vi "Inst_DS360.vi"(8 "error in":errorcluster, 10 "All Message Queues in":T1, 11 "Prueba08 in":refnum<class "Prueba08.lvclass">) -> (0 "error out":errorcluster)   [LabVIEW 2019, in "Prueba08.lvclass"]
uses:
  Prueba08.lvclass
  QMH/Message Queue/All Message Queues.ctl
  QMH/Message Queue/Message Cluster.ctl
  Prueba08.lvclass/Prueba08.ctl
  ClusterGEN.ctl
  <vilib>/Utility/error.llb/Error Cluster From Error Code.vi
  QMH/Message Queue/Enqueue Message (Single).vi
  <vilib>/ErrorRing/Error Ring.xnode
  QMH/Message Queue/Message Queue.lvlib
  Instrumento/DS360/DS360.lvclass
panel:
  out "All States":string[](array[string])
  out "Actual State":string
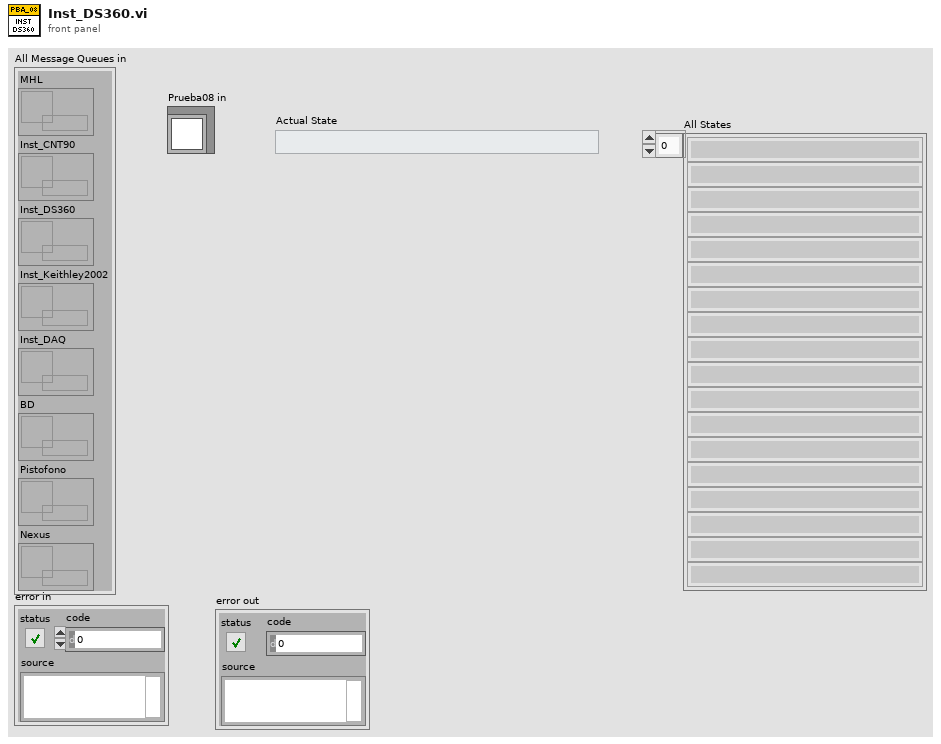
[diagram p1: front panel]
types:
  T1 = typedef "Message Queue.lvlib/All Message Queues.ctl" = cluster{"MHL":refnum<queue>, "Inst_CNT90":refnum<queue>, "Inst_DS360":refnum<queue>, "Inst_Keithley2002":refnum<queue>, "Inst_DAQ":refnum<queue>, "BD":refnum<queue>, "Pistofono":refnum<queue>, "Nexus":refnum<queue>}
  T2 = typedef "Prueba08.lvclass/ClusterGEN.ctl" = cluster{"frec":dbl, "amp":dbl, "ms_burst":dbl}
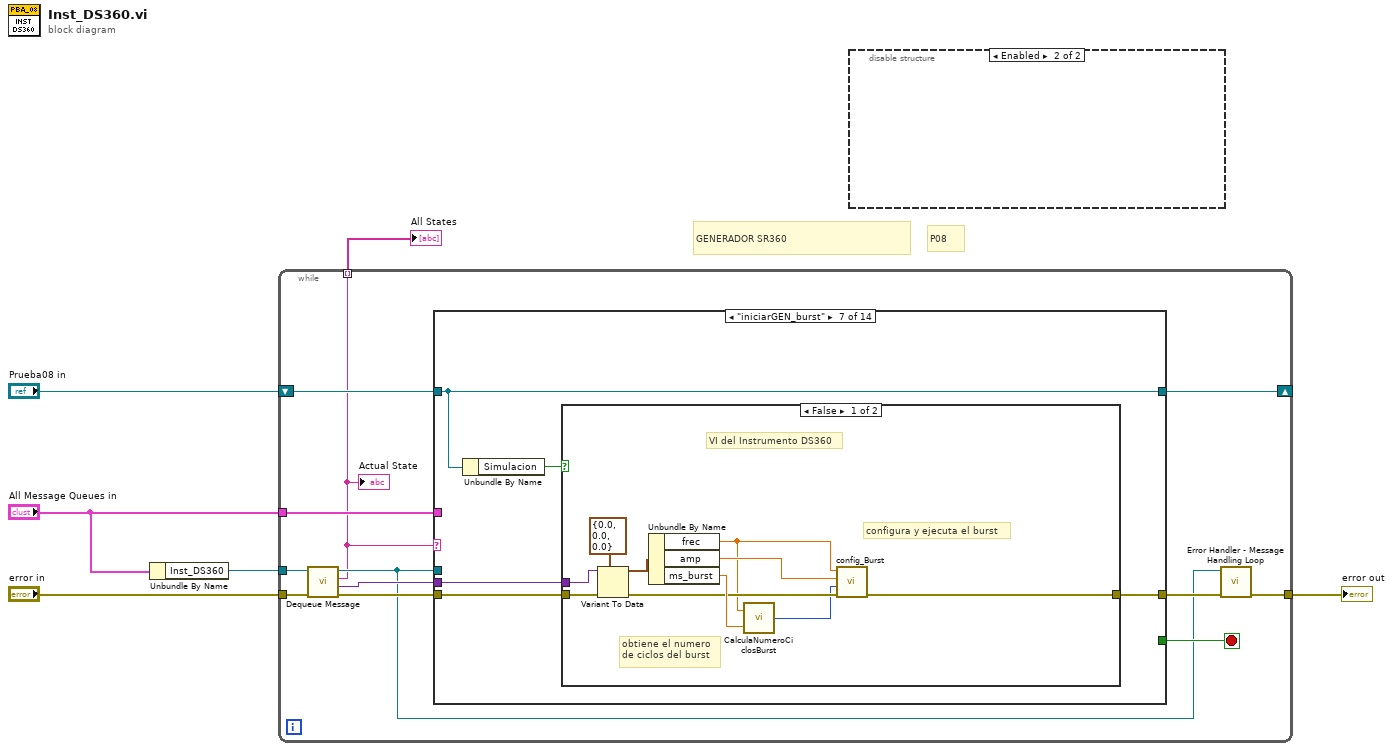
[diagram p0: block diagram]
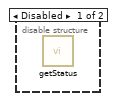
[diagram p2: hidden frame]
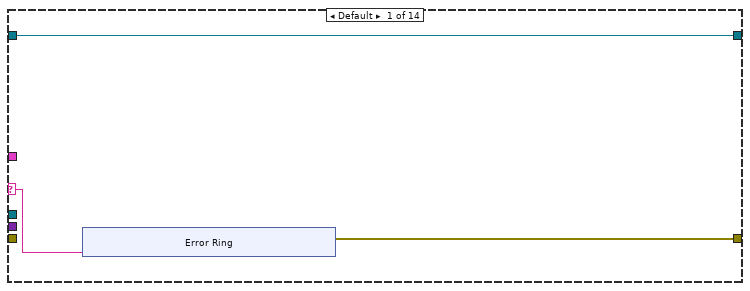
[diagram p3: hidden frame]
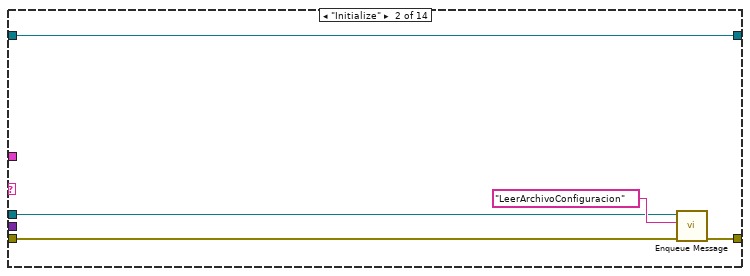
[diagram p4: hidden frame]
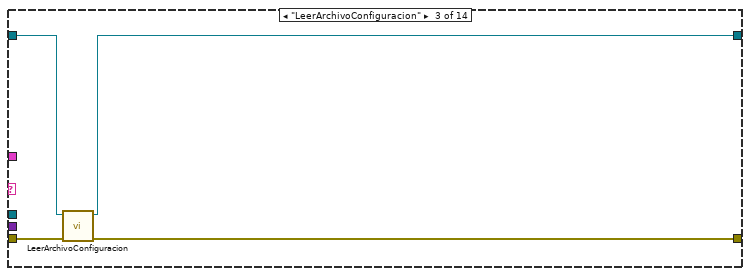
[diagram p5: hidden frame]
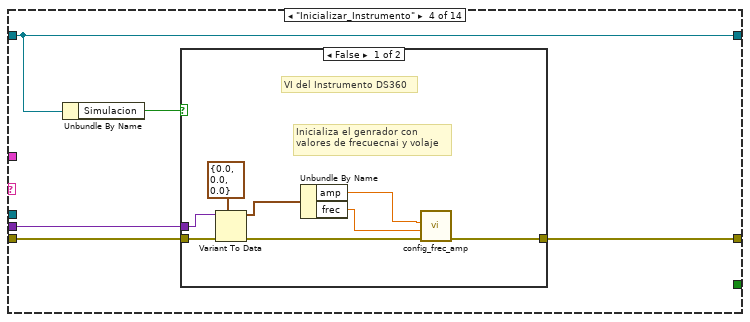
[diagram p6: hidden frame]
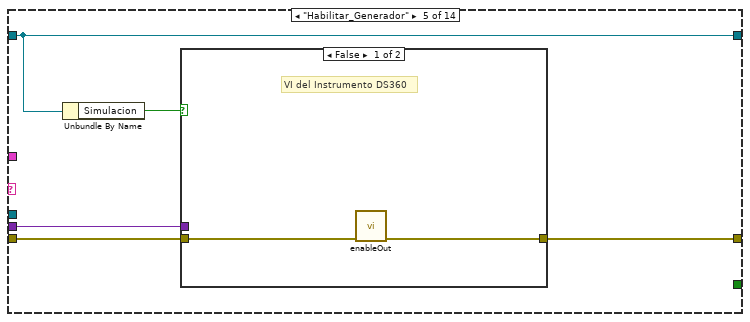
[diagram p8: hidden frame]
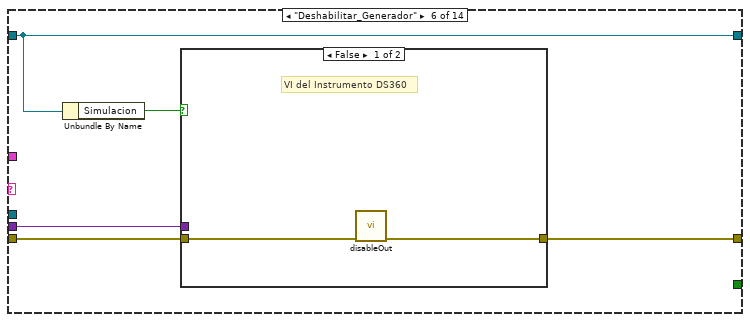
[diagram p10: hidden frame]
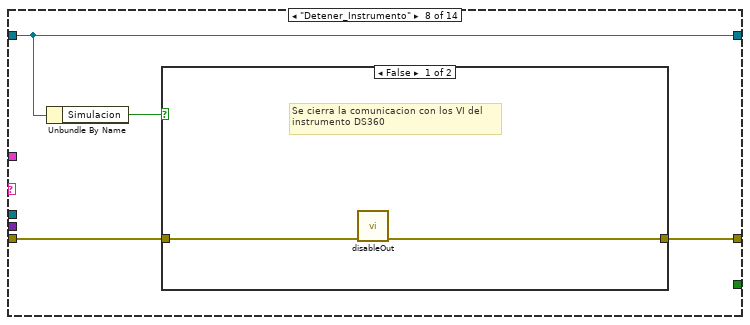
[diagram p13: hidden frame]
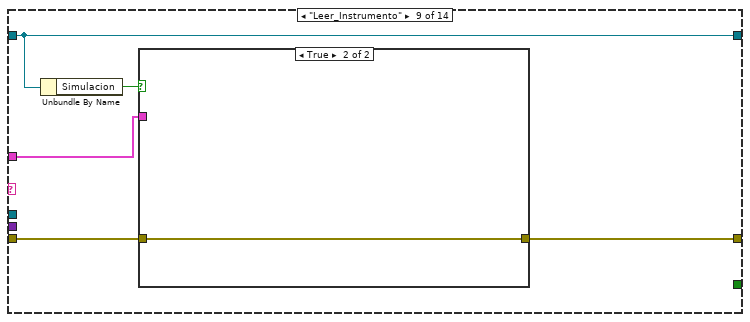
[diagram p15: hidden frame]
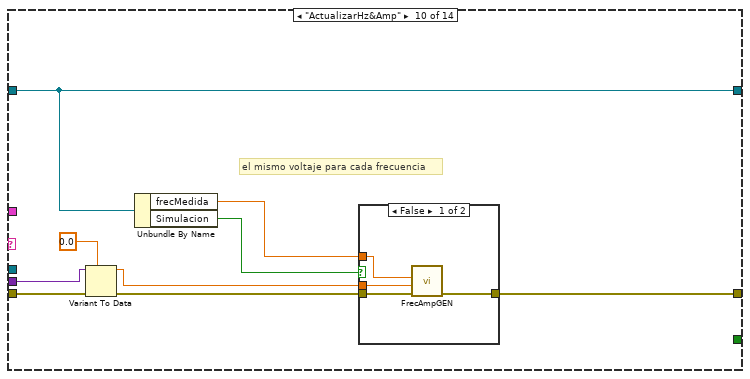
[diagram p17: hidden frame]
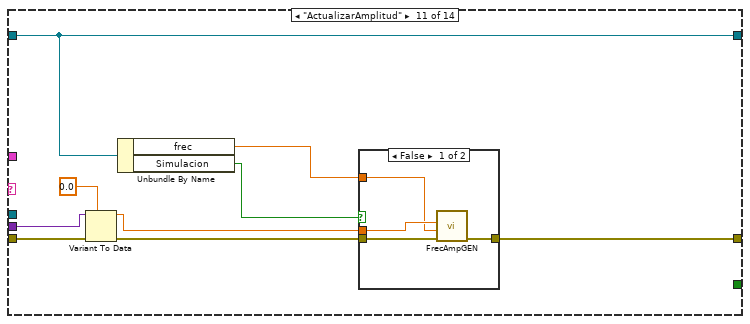
[diagram p19: hidden frame]
diagram:
  # "P08"
  # "GENERADOR SR360"
  n1 = Unbundle By Name("All Message Queues in") -> ("Inst_DS360"=w4:refnum<queue>)
  n2 = while {
    tunnel: "error in" -> [w18]
    tunnel: w4 -> [w17]
    tunnel: "All Message Queues in" -> [w16]
    tunnel: [w9] -> w2
    shift-right: [w12] -> _
    shift-left: "Prueba08 in" -> [w15]
    tunnel: [w7] -> w1 mode=indexing
    stop <- w11 stop-if-true
    n3 = call "Dequeue Message.vi"("error in (no error)"=w18, "Message Queue"=w17) -> ("error out"=w13:errorcluster, "Message Data"=w14:variant, "Message"=w7:string, "dup Message Queue"=w8:refnum<queue>)  [unwired: 6 in]
    "Actual State" <- w7
    n4 = case shown="\"iniciarGEN_burst\"" w7 {
      selector: w7 -> [w21 _ _ _ _ _ _ _ _ _ _ _ w140 _]
      tunnel: w16 -> [_ _ _ _ _ _ _ _ w94 _ _ _ w139 _]
      tunnel: w15 -> [w19 w33 w34 w40 w54 w62 w70 w86 w93 w102 w116 w129 w147 w149]
      tunnel: w8 -> [_ w29 _ _ _ _ _ _ _ _ _ _ _ w151]
      tunnel: w14 -> [_ _ _ w39 w53 w61 w69 _ _ w103 w117 w130 w144 _]
      tunnel: w13 -> [_ w30 w36 w38 w52 w60 w68 w84 w95 w104 w118 w131 w145 w152]
      tunnel: [w20 w31 w37 w42 w56 w64 w72 w87 w91 w106 w120 w133 w142 w148] -> w10
      tunnel: [w19 w33 w35 w40 w54 w62 w70 w86 w93 w102 w116 w129 w147 w149] -> w12
      tunnel: [_ _ _ _ _ _ _ _ _ _ _ _ _ TRUE] -> w11
      frame Default {
        n5 = xnode "Error Ring"("parameter 0"=w21) -> ("error out"=w20:errorcluster)
      }
      frame "Initialize" {
        n6 = call-poly "Enqueue Message.vi"("error in (no error)"=w30, "Message"="LeerArchivoConfiguracion", "Message Queue"=w29) -> ("error out"=w31:errorcluster)  [unwired: 7 in, 1 out]
      }
      frame "LeerArchivoConfiguracion" {
        n7 = call "LeerArchivoConfiguracion.vi"("error in"=w36, "Prueba31 in"=w34) -> ("error out"=w37:errorcluster, "Prueba31 out"=w35:refnum<class "Prueba08.lvclass">)  [unwired: 8 in]
      }
      frame "Inicializar_Instrumento" {
        n8 = Unbundle By Name(w40) -> ("Simulacion"=w41:bool)
        n9 = case shown="False" w41 {
          tunnel: [w49 w51] -> w42
          tunnel: w38 -> [w50 w51]
          tunnel: w39 -> [w47 _]
          frame False {
            # "Inicializa el genrador con \nvalores de frecuecnai y volaje"
            # "VI del Instrumento DS360"
            n10 = Variant To Data(error in=w50, type=T2 {"frec"=0.0, "amp"=0.0, "ms_burst"=0.0} ("clusterGEN"), Variant=w47) -> (data=w46:T2, error out=w48:errorcluster)
            n11 = Unbundle By Name(w46) -> ("amp"=w45:dbl, "frec"=w44:dbl)
            n12 = call "config_frec_amp.vi"("error in (no error)"=w48, "Frec (Hz)"=w44, "Amplitud (Vrms)"=w45) -> ("error out"=w49:errorcluster)  [unwired: 7 in, 1 out]
          }
          frame True {
            # "Simulacion"
          }
        }
      }
      frame "Habilitar_Generador" {
        n13 = Unbundle By Name(w54) -> ("Simulacion"=w55:bool)
        n14 = case shown="False" w55 {
          tunnel: [w57 w59] -> w56
          tunnel: w52 -> [w58 w59]
          tunnel: w53 -> [_ _]
          frame False {
            # "VI del Instrumento DS360"
            n15 = call "enableOut.vi"("error in (no error)"=w58) -> ("error out"=w57:errorcluster)  [unwired: 9 in, 1 out]
          }
          frame True {
            # "Simulacion"
          }
        }
      }
      frame "Deshabilitar_Generador" {
        n16 = Unbundle By Name(w62) -> ("Simulacion"=w63:bool)
        n17 = case shown="False" w63 {
          tunnel: [w65 w67] -> w64
          tunnel: w60 -> [w66 w67]
          tunnel: w61 -> [_ _]
          frame False {
            # "VI del Instrumento DS360"
            n18 = call "disableOut.vi"("error in (no error)"=w66) -> ("error out"=w65:errorcluster)  [unwired: 9 in, 1 out]
          }
          frame True {
            # "Simulacion"
          }
        }
      }
      frame "iniciarGEN_burst" {
        n19 = Unbundle By Name(w70) -> ("Simulacion"=w71:bool)
        n20 = case shown="False" w71 {
          tunnel: [w74 w83] -> w72
          tunnel: w68 -> [w82 w83]
          tunnel: w69 -> [w81 _]
          frame False {
            # "configura y ejecuta el burst"
            # "obtiene el numero\nde ciclos del burst"
            # "VI del Instrumento DS360"
            n21 = Variant To Data(error in=w82, type=T2 {"frec"=0.0, "amp"=0.0, "ms_burst"=0.0} ("clusterGEN"), Variant=w81) -> (data=w80:T2, error out=w77:errorcluster)
            n22 = Unbundle By Name(w80) -> ("frec"=w73:dbl, "amp"=w76:dbl, "ms_burst"=w78:dbl)
            n23 = call "CalculaNumeroCiclosBurst.vi"("ms_burst"=w78, "frec"=w73) -> ("# ciclos"=w75:i32)
            n24 = call "config_Burst.vi"("error in (no error)"=w77, "# ciclos"=w75, "Amplitud (Vrms)"=w76, "Frec (Hz)"=w73) -> ("error out"=w74:errorcluster)  [unwired: 6 in, 1 out]
          }
          frame True {
            # "Simulacion"
          }
        }
      }
      frame "Detener_Instrumento" {
        n25 = Unbundle By Name(w86) -> ("Simulacion"=w85:bool)
        n26 = case shown="False" w85 {
          tunnel: [w89 w90] -> w87
          tunnel: w84 -> [w88 w90]
          frame False {
            # "Se cierra la comunicacion con los VI del\ninstrumento DS360"
            n27 = call "disableOut.vi"("error in (no error)"=w88) -> ("error out"=w89:errorcluster)  [unwired: 9 in, 1 out]
          }
          frame True {
            # "Simulacion"
          }
        }
      }
      frame "Leer_Instrumento" {
        n28 = Unbundle By Name(w93) -> ("Simulacion"=w92:bool)
        n29 = case shown="True" w92 {
          tunnel: [w96 w97] -> w91
          tunnel: w95 -> [w96 w97]
          tunnel: w94 -> [_ _]
          frame False {
          }
          frame True {
          }
        }
      }
      frame "ActualizarHz&Amp" {
        # "el mismo voltaje para cada frecuencia"
        n30 = Variant To Data(error in=w104, type=0.0, Variant=w103) -> (data=w99:dbl, error out=w105:errorcluster)
        n31 = Unbundle By Name(w102) -> ("frecMedida"=w101:dbl, "Simulacion"=w98:bool)
        n32 = case shown="False" w98 {
          tunnel: [w110 w111] -> w106
          tunnel: w105 -> [w109 w111]
          tunnel: w101 -> [w108 _]
          tunnel: w99 -> [w107 _]
          frame False {
            n33 = call "FrecAmpGEN.vi"("error in (no error)"=w109, "Frec (Hz)"=w107, "Amplitud (Vrms)"=w108) -> ("error out"=w110:errorcluster)  [unwired: 7 in, 1 out]
          }
          frame True {
            # "Simlacion"
          }
        }
      }
      frame "ActualizarAmplitud" {
        n34 = Variant To Data(error in=w118, type=0.0, Variant=w117) -> (data=w114:dbl, error out=w119:errorcluster)
        n35 = Unbundle By Name(w116) -> ("frec"=w112:dbl, "Simulacion"=w113:bool)
        n36 = case shown="False" w113 {
          tunnel: [w124 w125] -> w120
          tunnel: w119 -> [w123 w125]
          tunnel: w114 -> [w122 _]
          tunnel: w112 -> [w121 _]
          frame False {
            n37 = call "FrecAmpGEN.vi"("error in (no error)"=w123, "Frec (Hz)"=w121, "Amplitud (Vrms)"=w122) -> ("error out"=w124:errorcluster)  [unwired: 7 in, 1 out]
          }
          frame True {
            # "Simlacion"
          }
        }
      }
      frame "ActualizarFrecuencia" {
        # "el mismo voltaje para cada frecuencia"
        n38 = Variant To Data(error in=w131, type=0.0, Variant=w130) -> (data=w127:dbl, error out=w132:errorcluster)
        n39 = Unbundle By Name(w129) -> ("Simulacion"=w126:bool)
        n40 = case shown="False" w126 {
          tunnel: [w136 w137] -> w133
          tunnel: w132 -> [w135 w137]
          tunnel: w127 -> [w134 _]
          frame False {
            n41 = call "FrecAmpGEN.vi"("error in (no error)"=w135, "Frec (Hz)"=w134) -> ("error out"=w136:errorcluster)  [unwired: 8 in, 1 out]
          }
          frame True {
            # "Simlacion"
          }
        }
      }
      frame "Error" {
        n42 = Unbundle By Name(w139) -> ("MHL"=w138:refnum<queue>)
        n43 = Variant To Data(error in=w145, type=errorcluster {"status"=FALSE, "code"=0, "source"=""} ("error constant"), Variant=w144) -> (data=w141:errorcluster, error out=w143:errorcluster)
        n44 = call-poly "Enqueue Message.vi"("error in (no error)"=w143, "Message Data"=w141, "Message"=w140, "Message Queue"=w138) -> ("error out"=w142:errorcluster)  [unwired: 6 in, 1 out]
      }
      frame "Exit" {
        n45 = Release Queue(queue=w151, error in (no error)=w152) -> (error out=w148:errorcluster)  [unwired: 1 in, 2 out]
      }
    }
    n46 = call "Error Handler - Message Handling Loop.vi"("error in (no error)"=w10, "Message Queue"=w8) -> ("dup error in"=w9:errorcluster)  [unwired: 8 in, 1 out]
  }
  "error out" <- w2
  "All States" <- w1
  n47 = disable-structure shown="Enabled" {
    frame Disabled {
      n48 = call "getStatus.vi"() -> ()  [unwired: 9 in, 3 out]
    }
    frame Enabled {
    }
  }
